vi "Copy .LLB to NI VeriStand dir.vi"(5 "Files Generated by Build":path[](array[path]), 6 "Top Level/Always Included VIs":path[](array[path]), 7 "Destination Path":path, 8 "error in (no error)":errorcluster, 9 "Target Name":string, 10 "Build Specification Name":string, 11 "Project Path":path) -> (0 "error out":errorcluster)   [LabVIEW 2017]
doc: "This VI is called after each run of a build specification. The VI will copy the generated LLB (Engine or System Explorer) into the VeriStand Custom Device folder (...\\Documents\\National Instruments\\NI VeriStand 2013...)."
uses:
  <vilib>/Utility/sysdir.llb/System Directory Type.ctl
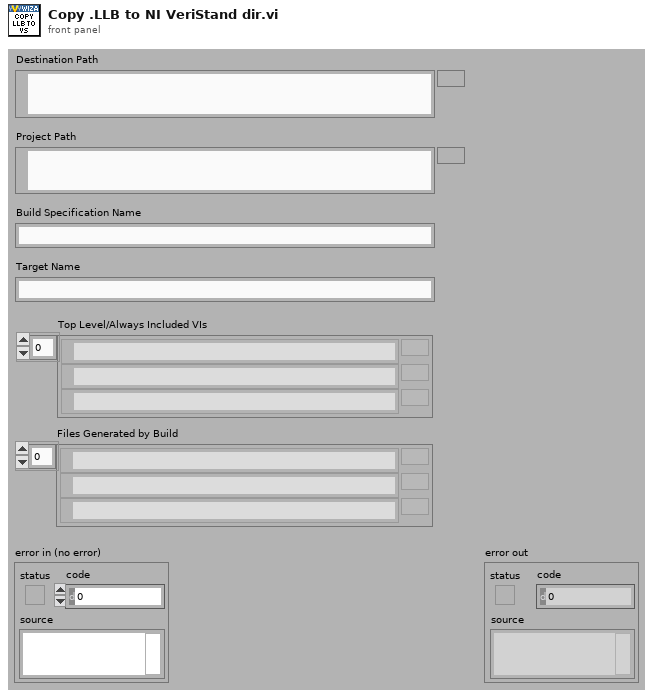
[diagram p1: front panel]
types:
  T1 = typedef "System Directory Type.ctl" = i32
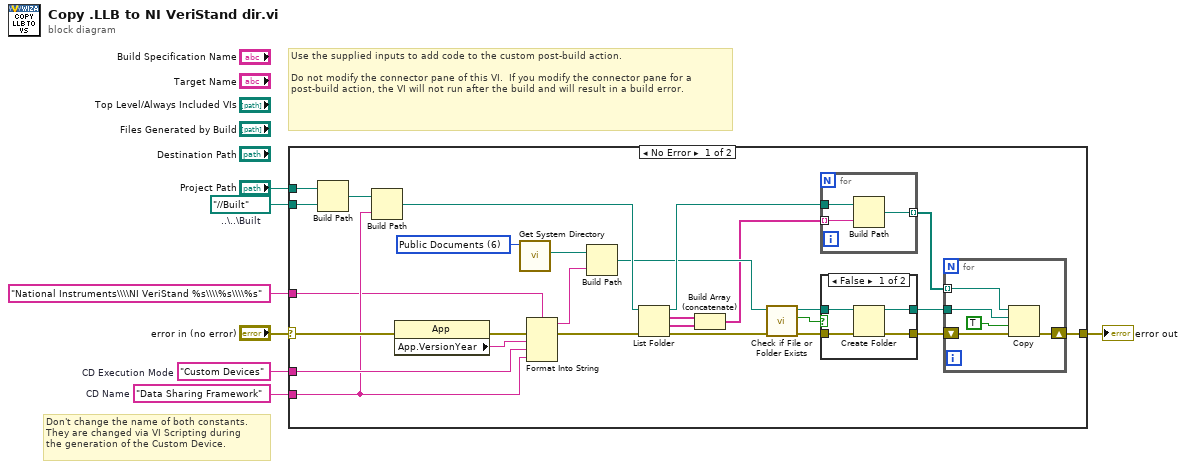
[diagram p0: block diagram]
diagram:
  w1 = path "../../Built"  # ..\..\Built
  w4 = "Data Sharing Framework"  # CD Name
  w5 = "Custom Devices"  # CD Execution Mode
  # "Use the supplied inputs to add code to the custom post-build action.\n\nDo not modify the connector pane of this VI.  If you modify the connector pane for a post-build action, the VI will not run after the build and will result in a build error."
  # "Don't change the name of both constants.\nThey are changed via VI Scripting during\nthe generation of the Custom Device."
  n1 = case shown="No Error" "error in (no error)" {
    selector: "error in (no error)" -> [w18 w49]
    tunnel: [w21 w49] -> w3
    tunnel: "Project Path" -> [w15 _]
    tunnel: w5 -> [w19 _]
    tunnel: w4 -> [w16 _]
    tunnel: "National Instruments\\\\NI VeriStand %s\\\\%s\\\\%s" ("name or relative path") -> [w9 _]
    tunnel: w1 -> [w8 _]
    frame No Error {
      w24 = T1 6 items=["User Home"=0, "User Desktop"=1, "User Documents"=2, "User Application Data"=3, "User Preferences"=4, "User Temporary"=5, "Public Documents"=6, "Public Application Data"=7, "Public Preferences"=8, "Public Cache"=13, "System Core Libraries"=9, "System Installed Libraries"=10, "Application Files"=11, "Boot Volume Root"=12] ("system directory type")
      n2 = Build Path(base path=w15, name or relative path=w8) -> (appended path=w27:path)
      n3 = Build Path(base path=w27, name or relative path=w16) -> (appended path=w29:path)
      n4 = property class="App"(error in=w18) -> (error out=w23:errorcluster, "App.VersionYear"=w22:string)  [unwired: 1 in, 1 out]
      n5 = call <vilib>:"Get System Directory.vi"("system directory type"=w24) -> ("system directory"=w25:path)  [unwired: 10 in]
      n6 = Format Into String(format string=w9, error in=w23, w22, w19, w16) -> (resulting string=w26:string, error out=w17:errorcluster)  [unwired: 1 in]
      n7 = Build Path(base path=w25, name or relative path=w26) -> (appended path=w20:path)
      n8 = List Folder(path=w29, error in=w17) -> (path out=w31:path, filenames=w12:string[], folder names=w11:string[], error out=w28:errorcluster)  [unwired: 2 in]
      n9 = Build Array (concatenate)(w12, w11) -> (w10:string[])
      n10 = call <vilib>:"Check if File or Folder Exists.vi"("error in (no error)"=w28, "path"=w20) -> ("error out"=w32:errorcluster, "file or folder exists?"=w34:bool, "dup path"=w33:path)  [unwired: 7 in]
      n11 = for {
        tunnel: w10 -> [w47] mode=indexing
        tunnel: w31 -> [w48]
        tunnel: [w46] -> w30 mode=indexing
        n12 = Build Path(base path=w48, name or relative path=w47) -> (appended path=w46:path)
      }
      n13 = case shown="False" w34 {
        tunnel: w33 -> [w38 w40]
        tunnel: w32 -> [w37 w39]
        tunnel: [w36 w40] -> w14
        tunnel: [w35 w39] -> w13
        frame False {
          n14 = Create Folder(path (use dialog)=w38, error in=w37) -> (created path=w36:path, error out=w35:errorcluster)  [unwired: 1 in, 1 out]
        }
        frame True {
        }
      }
      n15 = for {
        tunnel: w30 -> [w42] mode=indexing
        shift-right: [w43] -> w21
        shift-left: w13 -> [w44]
        tunnel: w14 -> [w41]
        n16 = Copy(8:w44, 9:TRUE ("overwrite (F)"), 10:w41, 11:w42) -> (0:w43:errorcluster)  [unwired: 1 in, 2 out]
      }
    }
    frame Error {
    }
  }
  "error out" <- w3
